vi "Autonomous Independent.vi"() -> ()   [LabVIEW 2019]
doc: "This VI is called when autonomous begins, and will automatically be terminated when autonomous ends. You can carry out timed or sensor driven robot movement independently without needing to return to the caller."
uses:
  <vilib>/Rock Robotics/WPI/ThirdParty/ADI/ADIS16448/Typedef/ADIS16448 Data.ctl
  <vilib>/Rock Robotics/WPI/ThirdParty/ADI/ADIS16448/Typedef/ADIS16448 Status.ctl
  <vilib>/Rock Robotics/WPI/Utilities/WPI_GetSetVariantRefNum.vi
  <vilib>/Rock Robotics/Network Tables/NT Read String.vi
  <vilib>/Rock Robotics/Network Tables/NT Write Numeric Array.vi
  <vilib>/Rock Robotics/WPI/RobotDrive/WPI_RobotDriveArcadeDrive_Standard(NoSaturation).vi
  <vilib>/addons/control/pid/NI_PID_pid.lvlib
  <vilib>/addons/control/pid/pid.llb/PID (DBL).vi
panel:
  out "dt out (s) 2":dbl format="%.3f"
  out "dt out (s)":dbl format="%.3f"
  in  "setpoint 2":dbl=90.0 format="%#_13g"
  in  "setpoint":dbl=300.0 format="%#_13g"
  out "ADIS16448 Status":T1
  out "Motor Values":dbl[](array[numeric])
  out "ADIS16448 Value":T2
  in  "PID gains 2":T3={"proportional gain (Kc)"=1.0, "integral time (Ti, min)"=0.0002, "derivative time (Td, min)"=0.01} {"derivative time (Td, min)" format="%.5f"; "integral time (Ti, min)" format="%.5f"; "proportional gain (Kc)" format="%.3f"}
  in  "PID gains":T4={"proportional gain (Kc)"=0.01, "integral time (Ti, min)"=0.0, "derivative time (Td, min)"=0.002} {"derivative time (Td, min)" format="%.3f"; "integral time (Ti, min)" format="%.3f"; "proportional gain (Kc)" format="%.3f"}
  out "Right":dbl
  out "Left":dbl
  out "Current Movement, for debugging":T5 {"Y Joystick Value" scale=1.0..-1.0; "X Joystick Value" scale=-1.0..1.0}
  in  "Array of robot movements":T6(array[cluster])=[{"X Joystick Value"=0.39393939393939403, "Y Joystick Value"=0.0, "Delay (sec)"=1.0, "Movement Name"="turn"}, {"X Joystick Value"=-0.3737373737373737, "Y Joystick Value"=0.0, "Delay (sec)"=1.0, "Movement Name"="turn back"}] {"Y Joystick Value" scale=1.0..-1.0; "X Joystick Value" scale=-1.0..1.0}
  # "Be sure to right-click and choose Data Operations>>Make Current Value default if you want to save the array values with the VI"
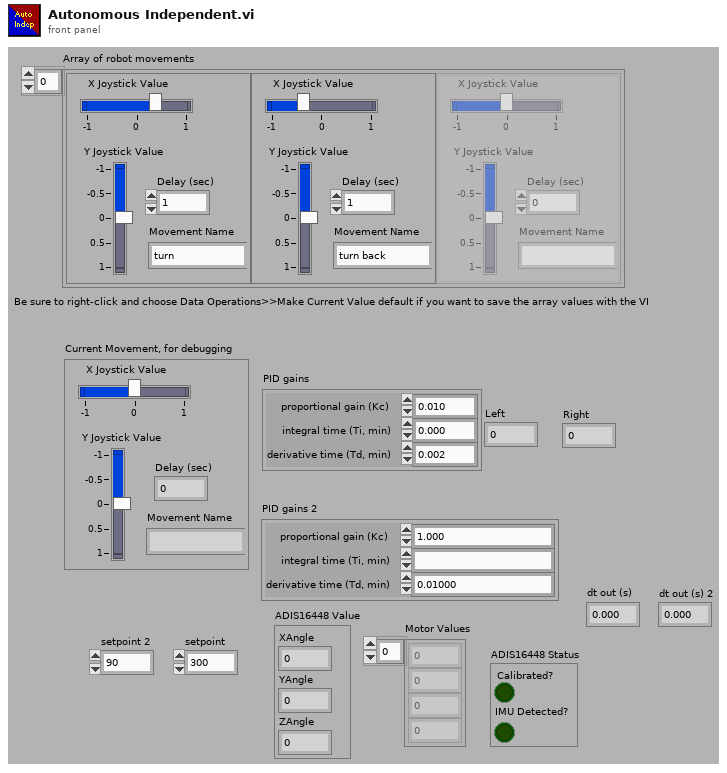
[diagram p1: front panel]
types:
  T1 = typedef "ADIS16448 Status.ctl" = cluster{"Calibrated?":bool, "IMU Detected?":bool}
  T2 = typedef "ADIS16448 Data.ctl" = cluster{"XAngle":dbl, "YAngle":dbl, "ZAngle":dbl}
  T3 = cluster{"proportional gain (Kc)":dbl, "integral time (Ti, min)":ext, "derivative time (Td, min)":dbl}
  T4 = cluster{"proportional gain (Kc)":dbl, "integral time (Ti, min)":dbl, "derivative time (Td, min)":dbl}
  T5 = cluster{"X Joystick Value":dbl, "Y Joystick Value":dbl, "Delay (sec)":dbl, "Movement Name":string}
  T6 = cluster{"X Joystick Value":dbl, "Y Joystick Value":dbl, "Delay (sec)":dbl, "Movement Name":string}[]
  T7 = typedef "WPI_JoystickDevRef.ctl" = cluster{"Device":T8}
  T8 = typedef "WPI_JoystickDeviceEnum.ctl" = enum16{"USB 0", "USB 1", "USB 2", "USB 3", "USB 4", "USB 5"}
  T9 = typedef "WPI_EncoderDevRef.ctl" = cluster{"DevStatus":errorcluster, "EncoderIndex":T10, "CounterIndex":T11, "DistancePerCount":dbl, "Decoding Type":T12}
  T10 = typedef "FPGA_EncoderIdx.ctl" = enum8{"Enc 0", "Enc 1", "Enc 2", "Enc 3", "Enc 4", "Enc 5", "Enc 6", "Enc 7", "Invalid"}
  T11 = typedef "FPGA_CounterCtrSystemIndex.ctl" = enum8{"Ctr 0", "Ctr 1", "Ctr 2", "Ctr 3", "Ctr 4", "Ctr 5", "Ctr 6", "Ctr 7", "Invalid"}
  T12 = typedef "WPI_EncoderType.ctl" = enum16{"1x", "2x", "4x"}
  T13 = typedef "ADIS16448 Device Reference.ctl" = cluster{"DevStatus":errorcluster, "Hardware Config":T14, "Calibration Complete":refnum<notifier>, "Status FIFO":refnum<k33>, "Last Value Reference":refnum<data-value>, "Sychronous Process VI":T18, "Cmd FIFO":refnum<k33>, "Source":T19, "Data FIFO":refnum<k33>, "IMU Status LED Pin":T16, "Calibration Time":u32}
  T14 = typedef "ADIS16448 Hardware Configuration.ctl" = cluster{"SPI Clock Rate (Hz)":dbl, "IMU SPI Mode (3)":T15, "IMU Reset Pin":T16, "IMU SPI Bus":T17, "IMU Data Ready Pin":T16, "Stall Config":cluster{"Pow2BytesPerRead":u8, "StallTicks":u16, "CsToSclkTicks":u8}, "IMU Status LED Pin":T16}
  T15 = typedef "WPI_SPIMode.ctl" = enum16{"Mode 0 (Clk Idle Low,Sample on Leading)", "Mode 1 (Clk Idle Low,Sample on Trailing)", "Mode 2 (Clk Idle High,Sample on Leading)", "Mode 3 (Clk Idle High,Sample on Trailing)"}
  T16 = typedef "FPGA_DIOChannel.ctl" = enum8{"DIO 0", "DIO 1", "DIO 2", "DIO 3", "DIO 4", "DIO 5", "DIO 6", "DIO 7", "DIO 8", "DIO 9", "DIO MXP 0", "DIO MXP 1", "DIO MXP 2", "DIO MXP 3", "DIO MXP 4", "DIO MXP 5", "DIO MXP 6", "DIO MXP 7", "DIO MXP 8", "DIO MXP 9", "DIO MXP 10", "DIO MXP 11", "DIO MXP 12", "DIO MXP 13", "DIO MXP 14", "DIO MXP 15", "SPI Port CS1", "SPI Port CS2", "SPI Port CS3", "SPI Port MISO", "SPI Port MOSI", "Invalid"}
  T17 = typedef "spi_bus.ctl" = enum16{"SPI On-Board, CS0", "SPI On-Board, CS1", "SPI On-Board, CS2", "SPI On-Board, CS3", "SPI MXP", "Invalid"}
  T18 = typedef "ADIS16448 Process.ctl" = refnum<vi>
  T19 = typedef "FPGA_CounterEncoderSourceConvertionLVSourceType.ctl" = cluster{"DevStatus":errorcluster, "AnalogTriggerMode?":bool, "DigitalMode":cluster{"DIO Channel":T20}, "AnalogTriggerMode":cluster{"AnalogTriggerIndex":T21, "OutputType":T22}}
  T20 = typedef "FPGA_DIODigitalSourceChannel.ctl" = enum8{"DIO 0", "DIO 1", "DIO 2", "DIO 3", "DIO 4", "DIO 5", "DIO 6", "DIO 7", "DIO 8", "DIO 9", "DIO MXP 0", "DIO MXP 1", "DIO MXP 2", "DIO MXP 3", "DIO MXP 4", "DIO MXP 5", "DIO MXP 6", "DIO MXP 7", "DIO MXP 8", "DIO MXP 9", "DIO MXP 10", "DIO MXP 11", "DIO MXP 12", "DIO MXP 13", "DIO MXP 14", "DIO MXP 15", "SPI Port CS1", "SPI Port CS2", "SPI Port CS3", "SPI Port MISO", "SPI Port MOSI", "Disabled"}
  T21 = typedef "FPGA_AnalogTriggerIndex.ctl" = enum8{"Trig 0", "Trig 1", "Trig 2", "Trig 3", "Trig 4", "Trig 5", "Trig 6", "Trig 7", "Invalid"}
  T22 = typedef "FPGA_AnalogTriggerOutType.ctl" = enum16{"InWindow", "TriggerState", "Rising", "Falling"}
  T23 = typedef "WPI_RobotDriveDevRef.ctl" = cluster{"DevStatus":errorcluster, "Motors[]":T24[], "Square Inputs":bool, "Max Output":dbl}
  T24 = typedef "WPI_MotorControlDeviceRef.ctl" = cluster{"DeviceStatus":errorcluster, "Type":T25, "PWM":cluster{"PWM Channel":T26, "DeadBand":T27}, "CAN":cluster{"Device Number":u8, "SetOutput VI Ref":variant, "GetOutput VI Ref":variant, "Enable VI Ref":variant, "Disable VI Ref":variant, "Data":variant}, "Invert":bool, "DIO PWM":cluster{"PWM \"Enable\" Channel":T26, "DIOChannel":T16, "PWM Rate":dbl}}
  T25 = typedef "WPI_MotorControlType.ctl" = enum16{"PWM", "CAN", "DIO PWM"}
  T26 = typedef "FPGA_DIOPWMChannel.ctl" = enum8{"PWM 0", "PWM 1", "PWM 2", "PWM 3", "PWM 4", "PWM 5", "PWM 6", "PWM 7", "PWM 8", "PWM 9", "PWM MXP 0", "PWM MXP 1", "PWM MXP 2", "PWM MXP 3", "PWM MXP 4", "PWM MXP 5", "PWM MXP 6", "PWM MXP 7", "PWM MXP 8", "PWM MXP 9", "Invalid"}
  T27 = typedef "WPI_PWMDeadband.ctl" = cluster{"Name":string, "maxPositivePwm":i32, "minPositivePwm":i32, "centerPwm":i32, "maxNegativePwm":i32, "minNegativePwm":i32, "angularRange":u16}
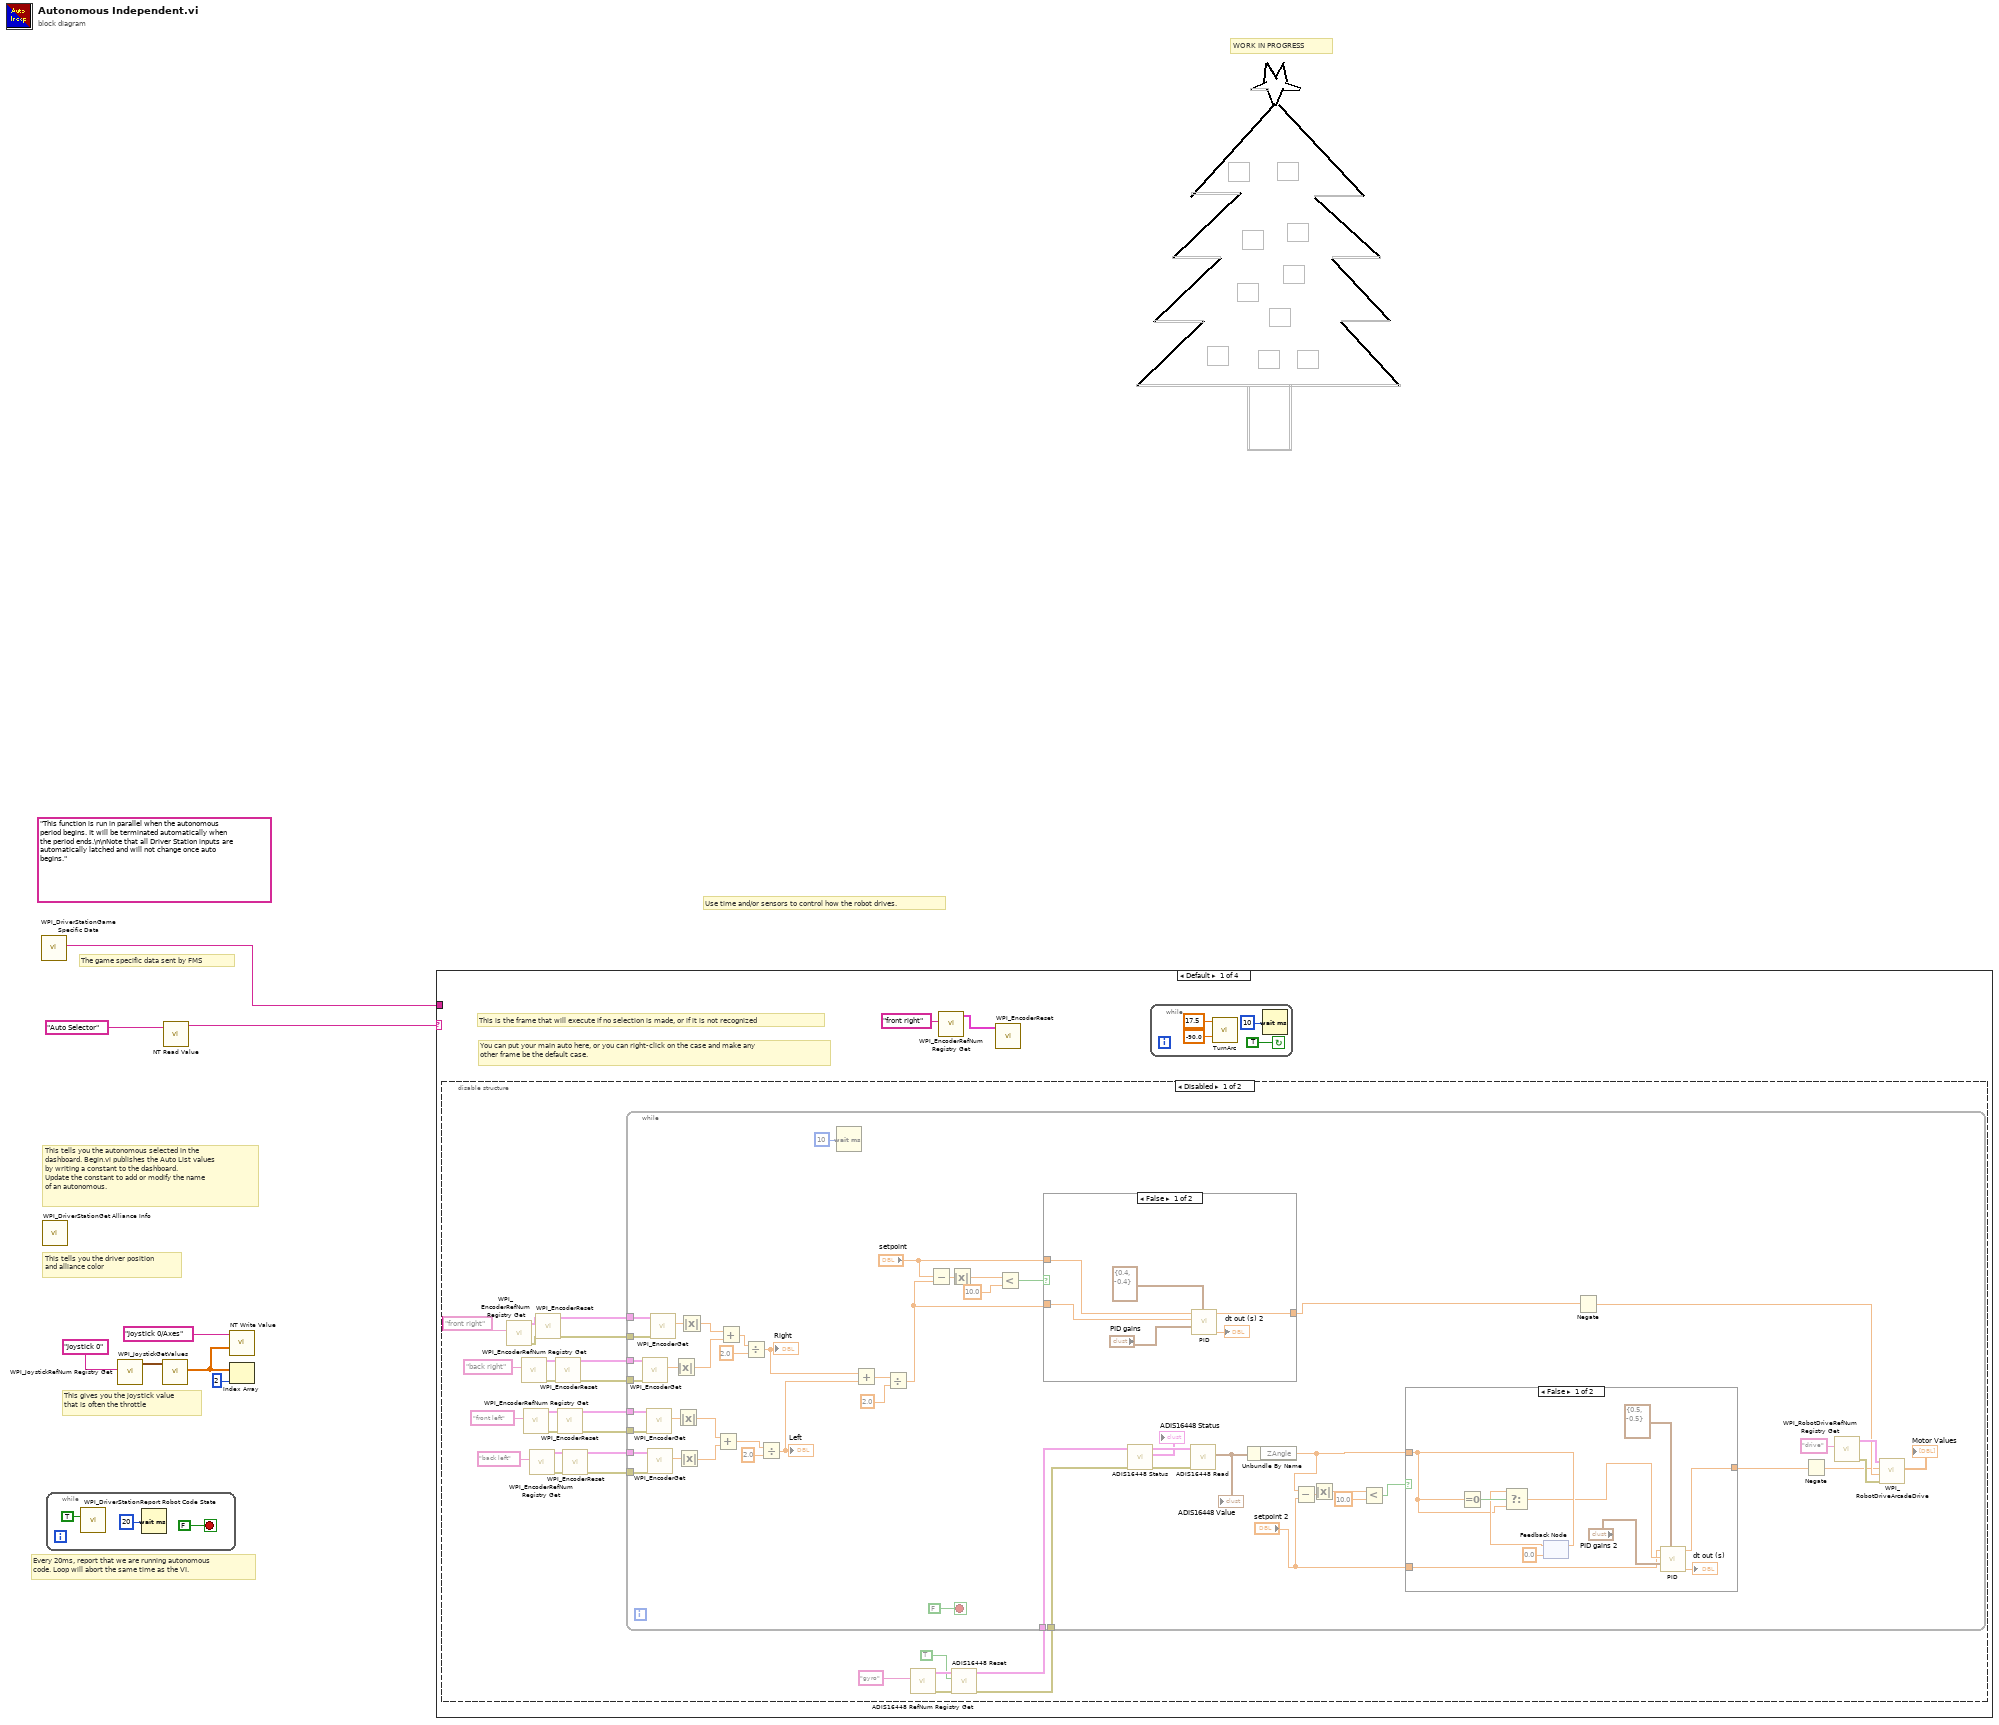
[diagram p0: block diagram]
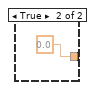
[diagram p2: hidden frame]
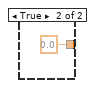
[diagram p3: hidden frame]
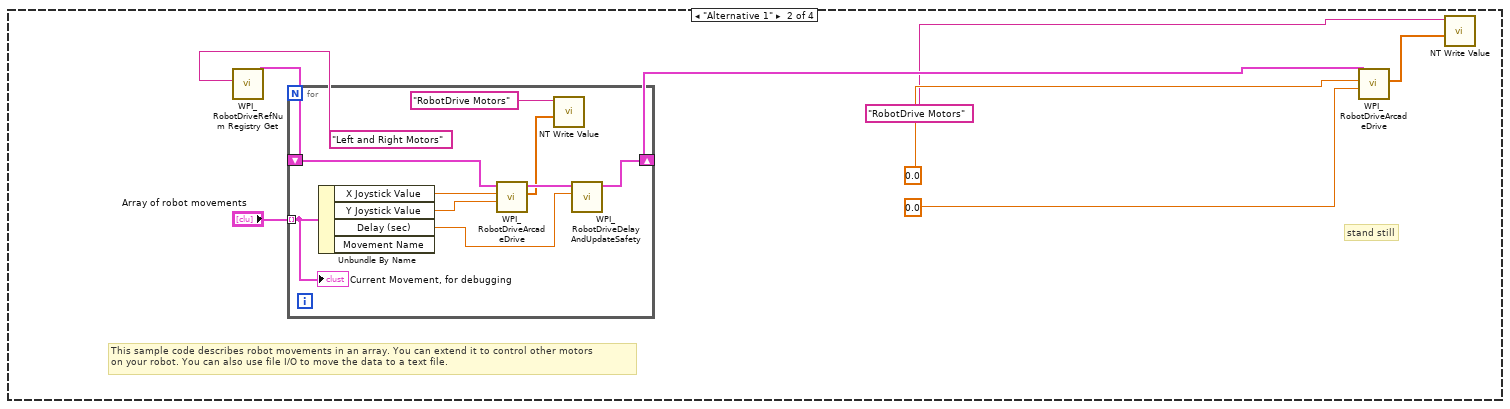
[diagram p5: hidden frame]
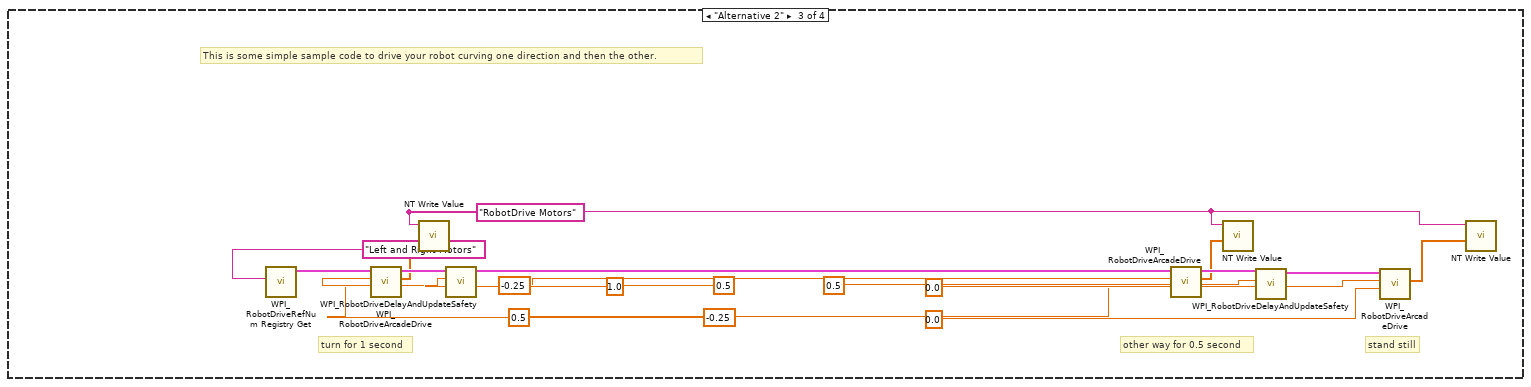
[diagram p6: hidden frame]
diagram:
  (unwired) "This function is run in parallel when the autonomous period begins. It will be terminated automatically when the period ends.\n\nNote that all Driver Station inputs are automatically latched and will not change once auto begins."
  # "WORK IN PROGRESS"
  # "The game specific data sent by FMS"
  # "This tells you the autonomous selected in the \ndashboard. Begin.vi publishes the Auto List values\nby writing a constant to the dashboard.\nUpdate the constant to add or modify the name\nof an autonomous."
  # "Every 20ms, report that we are running autonomous\ncode. Loop will abort the same time as the VI."
  # "This gives you the joystick value\nthat is often the throttle"
  # "Use time and/or sensors to control how the robot drives."
  # "This tells you the driver position\nand alliance color"
  n1 = call <vilib>:"WPI_DriverStationGame Specific Data.vi"() -> ("Game Specific Data"=w1:string)  [unwired: 11 in]
  n2 = call <vilib>:"WPI_DriverStationGet Alliance Info.vi"() -> ()  [unwired: 12 out]
  n3 = while {
    stop <- FALSE stop-if-true
    n4 = call <vilib>:"WPI_DriverStationReport Robot Code State.vi"("Autonomous"=TRUE) -> ()  [unwired: 10 in, 1 out]
    n5 = Wait (ms)(milliseconds to wait=u32 20) -> ()  [unwired: 1 out]
  }
  n6 = call <vilib>:"WPI_JoystickRefNum Registry Get.vi"("refnum name"="Joystick 0") -> ("JoystickDevRef"=w7:T7)  [unwired: 1 in, 9 out]
  n7 = call <vilib>:"WPI_JoystickGetValues.vi"("JoystickDevRef"=w7) -> ("Axes"=w3:dbl[])  [unwired: 6 in, 4 out]
  n8 = call-poly <vilib>:"NT Read Value.vi"("Name"="Auto Selector") -> ("String"=w4:string)  [unwired: 9 in, 1 out]
  n9 = call-poly <vilib>:"NT Write Value.vi"("Numeric Array"=w3, "Name"="Joystick 0/Axes") -> ()  [unwired: 9 in, 1 out]
  n10 = Index Array(array=w3, index=2) -> ()  [unwired: 1 out]
  n11 = case shown="Default" w4 {
    tunnel: w1 -> [_ _ _ _]
    frame Default {
      # "You can put your main auto here, or you can right-click on the case and make any\nother frame be the default case."
      # "This is the frame that will execute if no selection is made, or if it is not recognized"
      n12 = disable-structure shown="Disabled" {
        frame Disabled {
          n13 = call <vilib>:"WPI_EncoderRefNum Registry Get.vi"("refnum name"="front right") -> ("error out"=w26:errorcluster, "EncoderDevRef"=w27:T9)  [unwired: 9 in]
          n14 = call <vilib>:"WPI_EncoderRefNum Registry Get.vi"("refnum name"="back right") -> ("error out"=w28:errorcluster, "EncoderDevRef"=w29:T9)  [unwired: 9 in]
          n15 = call <vilib>:"WPI_EncoderRefNum Registry Get.vi"("refnum name"="front left") -> ("error out"=w30:errorcluster, "EncoderDevRef"=w31:T9)  [unwired: 9 in]
          n16 = call <vilib>:"WPI_EncoderRefNum Registry Get.vi"("refnum name"="back left") -> ("error out"=w32:errorcluster, "EncoderDevRef"=w33:T9)  [unwired: 9 in]
          n17 = call <vilib>:"WPI_EncoderReset.vi"("error in (no error)"=w26, "EncoderDevRef"=w27) -> ("error out"=w19:errorcluster, "EncoderDevRef"=w18:T9)  [unwired: 8 in]
          n18 = call <vilib>:"WPI_EncoderReset.vi"("error in (no error)"=w28, "EncoderDevRef"=w29) -> ("error out"=w21:errorcluster, "EncoderDevRef"=w20:T9)  [unwired: 8 in]
          n19 = call <vilib>:"WPI_EncoderReset.vi"("error in (no error)"=w30, "EncoderDevRef"=w31) -> ("error out"=w23:errorcluster, "EncoderDevRef"=w22:T9)  [unwired: 8 in]
          n20 = call <vilib>:"WPI_EncoderReset.vi"("error in (no error)"=w32, "EncoderDevRef"=w33) -> ("error out"=w25:errorcluster, "EncoderDevRef"=w24:T9)  [unwired: 8 in]
          n21 = call <vilib>:"ADIS16448 RefNum Registry Get.vi"("refnum name"="gyro") -> ("error out"=w43:errorcluster, "ADIS16448DevRef Out"=w42:T13)  [unwired: 9 in]
          n22 = call <vilib>:"ADIS16448 Reset.vi"("error in (no error)"=w43, "Reset?"=TRUE, "ADIS16448DevRef"=w42) -> ("error out"=w39:errorcluster, "ADIS16448DevRef"=w38:T13)  [unwired: 7 in]
          n23 = while {
            tunnel: w39 -> [w83]
            tunnel: w38 -> [w82]
            tunnel: w25 -> [w59]
            tunnel: w24 -> [w58]
            tunnel: w23 -> [w55]
            tunnel: w22 -> [w54]
            tunnel: w21 -> [w51]
            tunnel: w20 -> [w50]
            tunnel: w19 -> [w47]
            tunnel: w18 -> [w46]
            stop <- FALSE stop-if-true
            n24 = call <vilib>:"WPI_EncoderGet.vi"("error in (no error)"=w51, "EncoderDevRef"=w50) -> ("Distance"=w52:dbl)  [unwired: 4 in, 5 out]
            n25 = call <vilib>:"WPI_EncoderGet.vi"("error in (no error)"=w55, "EncoderDevRef"=w54) -> ("Distance"=w56:dbl)  [unwired: 4 in, 5 out]
            n26 = call <vilib>:"WPI_EncoderGet.vi"("error in (no error)"=w59, "EncoderDevRef"=w58) -> ("Distance"=w60:dbl)  [unwired: 4 in, 5 out]
            n27 = call <vilib>:"WPI_EncoderGet.vi"("error in (no error)"=w47, "EncoderDevRef"=w46) -> ("Distance"=w48:dbl)  [unwired: 4 in, 5 out]
            n28 = Absolute Value(x=w52) -> (abs(x)=w49:dbl)
            n29 = Absolute Value(x=w56) -> (abs(x)=w53:dbl)
            n30 = Absolute Value(x=w60) -> (abs(x)=w57:dbl)
            n31 = Absolute Value(x=w48) -> (abs(x)=w45:dbl)
            n32 = Add(x=w53, y=w57) -> (x+y=w93:dbl)
            n33 = Add(x=w45, y=w49) -> (x+y=w95:dbl)
            n34 = Divide(x=w95, y=2.0) -> (x/y=w88:dbl)
            "Right" <- w88
            n35 = Divide(x=w93, y=2.0) -> (x/y=w89:dbl)
            "Left" <- w89
            n36 = Wait (ms)(milliseconds to wait=u32 10) -> ()  [unwired: 1 out]
            n37 = Add(x=w88, y=w89) -> (x+y=w77:dbl)
            n38 = Divide(x=w77, y=2.0) -> (x/y=w74:dbl)
            n39 = Subtract(x="setpoint", y=w74) -> (x-y=w73:dbl)
            n40 = Absolute Value(x=w73) -> (abs(x)=w64:dbl)
            n41 = Less?(x=w64, y=10.0) -> (x < y?=w71:bool)
            n42 = case shown="False" w71 {
              tunnel: w74 -> [w110 _]
              tunnel: [w109 0.0 ("output")] -> w62
              tunnel: "setpoint" -> [w108 _]
              frame False {
                n43 = call-poly <vilib>:"PID.vi"("output range"=cluster{"output high":dbl, "output low":dbl} {"output high"=0.4, "output low"=-0.4}, "PID gains"="PID gains", "process variable"=w110, "setpoint"=w108) -> ("dt out (s)"=→"dt out (s) 2":dbl, "output"=w109:dbl)  [unwired: 6 in]
              }
              frame True {
              }
            }
            n44 = call <vilib>:"ADIS16448 Status.vi"("error in (no error)"=w83, "ADIS16448DevRef"=w82) -> ("error out"=w85:errorcluster, "ADIS16448 Status"=→"ADIS16448 Status":T1, "ADIS16448DevRef"=w86:T13)  [unwired: 7 in]
            n45 = call <vilib>:"ADIS16448 Read.vi"("error in (no error)"=w85, "ADIS16448DevRef"=w86) -> ("ADIS16448 Value"=w87:T2)  [unwired: 6 in, 3 out]
            "ADIS16448 Value" <- w87
            n46 = Unbundle By Name(w87) -> ("ZAngle"=w68:dbl)
            n47 = Subtract(x=w68, y="setpoint 2") -> (x-y=w70:dbl)
            n48 = Absolute Value(x=w70) -> (abs(x)=w65:dbl)
            n49 = Less?(x=w65, y=10.0) -> (x < y?=w66:bool)
            n50 = case shown="False" w66 {
              tunnel: w68 -> [w103 _]
              tunnel: [w98 0.0 ("output")] -> w61
              tunnel: "setpoint 2" -> [w97 _]
              frame False {
                n51 = Equal To 0?(x=w103) -> (x = 0?=w105:bool)
                n52 = feedback #1(0.0 ("ZAngle")) -> (w104:dbl)
                n53 = Select(t=w104, s=w105, f=w103) -> (s? t:f=w100:dbl)
                n54 = feedback-in #1(w103) -> ()
                n55 = call-poly <vilib>:"PID.vi"("output range"=cluster{"output high":dbl, "output low":dbl} {"output high"=0.5, "output low"=-0.5}, "PID gains"="PID gains 2", "process variable"=w100, "setpoint"=w97) -> ("dt out (s)"=→"dt out (s)":dbl, "output"=w98:dbl)  [unwired: 6 in]
              }
              frame True {
              }
            }
            n56 = Negate(x=w62) -> (-x=w63:dbl)
            n57 = Negate(x=w61) -> (-x=w44:dbl)
            n58 = call <vilib>:"WPI_RobotDriveRefNum Registry Get.vi"("refnum name"="drive") -> ("error out"=w79:errorcluster, "RobotDriveDevRef"=w81:T23)  [unwired: 9 in]
            n59 = call-poly <vilib>:"WPI_RobotDriveArcadeDrive.vi"("error in (no error)"=w79, "Y axis value"=w63, "X axis value"=w44, "RobotDriveDevRef"=w81) -> ("Motor Values"=→"Motor Values":dbl[])  [unwired: 5 in, 2 out]
          }
        }
        frame Enabled {
        }
      }
      n60 = call <vilib>:"WPI_EncoderRefNum Registry Get.vi"("refnum name"="front right") -> ("EncoderDevRef"=w13:T9)  [unwired: 9 in, 1 out]
      n61 = call <vilib>:"WPI_EncoderReset.vi"("EncoderDevRef"=w13) -> ()  [unwired: 9 in, 2 out]
      n62 = while {
        stop <- TRUE continue-if-true
        n63 = call "TurnArc.vi"("angle"=-90.0, "radius"=17.5) -> ()  [unwired: 10 in]
        n64 = Wait (ms)(milliseconds to wait=u32 10) -> ()  [unwired: 1 out]
      }
    }
    frame "Alternative 1" {
      # "stand still"
      # "This sample code describes robot movements in an array. You can extend it to control other motors\non your robot. You can also use file I/O to move the data to a text file."
      n65 = call <vilib>:"WPI_RobotDriveRefNum Registry Get.vi"("refnum name"="Left and Right Motors") -> ("RobotDriveDevRef"=w120:T23)  [unwired: 1 in, 9 out]
      n66 = for {
        shift-right: [w128] -> w115
        shift-left: w120 -> [w129]
        tunnel: "Array of robot movements" -> [w124] mode=indexing
        n67 = Unbundle By Name(w124) -> ("X Joystick Value"=w127:dbl, "Y Joystick Value"=w126:dbl, "Delay (sec)"=w125:dbl)  [unwired: 1 out]
        n68 = call-poly <vilib>:"WPI_RobotDriveArcadeDrive.vi"("Y axis value"=w126, "X axis value"=w127, "RobotDriveDevRef"=w129) -> ("Motor Values"=w122:dbl[], "RobotDriveDevRef"=w130:T23)  [unwired: 1 in, 6 out]
        n69 = call-poly <vilib>:"NT Write Value.vi"("Numeric Array"=w122, "Name"="RobotDrive Motors") -> ()  [unwired: 9 in, 1 out]
        n70 = call <vilib>:"WPI_RobotDriveDelayAndUpdateSafety.vi"("Delay (s)"=w125, "RobotDriveDevRef"=w130) -> ("RobotDriveDevRef 2"=w128:T23)  [unwired: 8 in, 1 out]
        "Current Movement, for debugging" <- w124
      }
      n71 = call-poly <vilib>:"WPI_RobotDriveArcadeDrive.vi"("Y axis value"=0.0 ("X axis value"), "X axis value"=0.0, "RobotDriveDevRef"=w115) -> ("Motor Values"=w118:dbl[])  [unwired: 1 in, 7 out]
      n72 = call-poly <vilib>:"NT Write Value.vi"("Numeric Array"=w118, "Name"="RobotDrive Motors") -> ()  [unwired: 9 in, 1 out]
    }
    frame "Alternative 2" {
      w132 = "RobotDrive Motors" ("Name")
      # "This is some simple sample code to drive your robot curving one direction and then the other."
      # "stand still"
      # "other way for 0.5 second"
      # "turn for 1 second"
      n73 = call <vilib>:"WPI_RobotDriveRefNum Registry Get.vi"("refnum name"="Left and Right Motors") -> ("RobotDriveDevRef"=w148:T23)  [unwired: 1 in, 9 out]
      n74 = call-poly <vilib>:"WPI_RobotDriveArcadeDrive.vi"("Y axis value"=0.5 ("X axis value"), "X axis value"=-0.25, "RobotDriveDevRef"=w148) -> ("Motor Values"=w131:dbl[], "RobotDriveDevRef"=w141:T23)  [unwired: 1 in, 6 out]
      n75 = call-poly <vilib>:"NT Write Value.vi"("Numeric Array"=w131, "Name"=w132) -> ()  [unwired: 9 in, 1 out]
      n76 = call <vilib>:"WPI_RobotDriveDelayAndUpdateSafety.vi"("Delay (s)"=1.0, "RobotDriveDevRef"=w141) -> ("RobotDriveDevRef 2"=w142:T23)  [unwired: 8 in, 1 out]
      n77 = call-poly <vilib>:"WPI_RobotDriveArcadeDrive.vi"("Y axis value"=-0.25 ("X axis value"), "X axis value"=0.5, "RobotDriveDevRef"=w142) -> ("Motor Values"=w133:dbl[], "RobotDriveDevRef"=w143:T23)  [unwired: 1 in, 6 out]
      n78 = call-poly <vilib>:"NT Write Value.vi"("Numeric Array"=w133, "Name"=w132) -> ()  [unwired: 9 in, 1 out]
      n79 = call <vilib>:"WPI_RobotDriveDelayAndUpdateSafety.vi"("Delay (s)"=0.5, "RobotDriveDevRef"=w143) -> ("RobotDriveDevRef 2"=w144:T23)  [unwired: 8 in, 1 out]
      n80 = call-poly <vilib>:"WPI_RobotDriveArcadeDrive.vi"("Y axis value"=0.0 ("X axis value"), "X axis value"=0.0, "RobotDriveDevRef"=w144) -> ("Motor Values"=w134:dbl[])  [unwired: 1 in, 7 out]
      n81 = call-poly <vilib>:"NT Write Value.vi"("Numeric Array"=w134, "Name"=w132) -> ()  [unwired: 9 in, 1 out]
    }
    frame "Your Turn" {
    }
  }
